vi "Main.vi"() -> ()   [LabVIEW 2017]
uses:
  <vilib>/Platform/TimedLoop/XDataNode/timing_clust.ctl
  <vilib>/Platform/TimedLoop/XDataNode/nitl_modes.ctl
  <vilib>/Platform/TimedLoop/XDataNode/wakeup.ctl
  <vilib>/Analysis/Matrix/Datatypes/RealMatrix.ctl
  <vilib>/Analysis/baseanly.llb/A x Vector.vi
  <vilib>/Analysis/baseanly.llb/Real A x B.vi
  <vilib>/Analysis/_algsub.llb/Real Vector Norm.vi
  <vilib>/Analysis/baseanly.llb/Outer Product.vi
  <vilib>/Analysis/baseanly.llb/Real Outer Product.vi
  <vilib>/robotics/Kinematics/Create Lie Group Matrix.vi
  <vilib>/Analysis/7linalg.llb/Create Special Matrix.vi
  <vilib>/Analysis/7linalg.llb/Create Special Real Matrix.vi
  <vilib>/Analysis/Matrix/Numeric/Multiply/Multiply.vi
  <vilib>/Analysis/Matrix/Numeric/Multiply/Multiply - RM,R.vi
  <vilib>/Analysis/Matrix/Numeric/Multiply/Multiply - R,RM.vi
  <vilib>/Analysis/Matrix/Numeric/Add/Add.vi
  <vilib>/Analysis/Matrix/Numeric/Add/Add - RM,RM.vi
  <vilib>/platform/TimedLoop/XDataNode/XDataNode.xnode
  <vilib>/robotics/Kinematics/NI_Kinematics.lvlib
  <vilib>/Analysis/NI_AALBase.lvlib
  <vilib>/Platform/TimedLoop/XDataNode/XDNodeRunTimeDep.lvlib
  <vilib>/Native 3D Graph/xcontrol/3DPC_SurfacePlot.xctl
  <vilib>/Analysis/Matrix/NI_Matrix.lvlib
  <vilib>/Analysis/NI_AALPro.lvlib
  <vilib>/Native 3D Graph/classes/Base Datatype.lvclass
panel:
  out "policy":dbl[](array[numeric])=[0.3333333333333333, 0.3333333333333333, 0.3333333333333333, 0.3333333333333333, 0.3333333333333333, 0.3333333333333333, 0.3333333333333333, 0.3333333333333333, 0.3333333333333333]
  out "w":dbl[][](array[numeric])
  out "theta":dbl[][](array[numeric])
  out "score":dbl=9.98
  out "break":bool=TRUE
  out "state":dbl[](array[numeric])=[1.3972445388219286, 0.08038206342090427, -148.25832903348876]
  in  "rom":dbl=-45.0
  out "rpy":dbl[](array[numeric])=[inf, inf, inf] format="%#_15g"
  in  "inertia":dbl=1.0
  out "torque":dbl[](array[numeric])
  in  "radius":dbl=1.0
  in  "damping":dbl=0.5
  out "beta2":dbl=0.7460127831658564
  out "v30":dbl[](array[numeric])=[0.5877852522924729, -0.33935797363675174, -0.7344008870614411]
  out "v10":dbl[](array[numeric])=[0.0, 0.6787159472735029, -0.7344008870614411]
  out "v20":dbl[](array[numeric])=[-0.5877852522924731, -0.3393579736367513, -0.7344008870614411]
  out "dt":dbl=0.001
  in  "period":i64=1
  out "v2":dbl[](array[numeric])=[-0.5834154431047975, -0.3393579736367513, -0.7378770808718702]
  out "v1":dbl[](array[numeric])=[0.004359453232169501, 0.6787159472735029, -0.7343879479431492]
  out "v3":dbl[](array[numeric])=[0.5921343495691362, -0.33935797363675174, -0.7308988150144282]
  out "theta":dbl[](array[numeric])=[0.004396877373720295, -0.002202197020422642, -0.002194719520146542] format="%#_15g"
  in  "stop":bool
  out "beta1":dbl=0.9553166181245093
  out "gamma2":dbl=1.2566370614359172
  out "gamma1":dbl=1.5707963267948966
  out "alpha2":dbl=1.5707963267948966
  out "alpha1":dbl=1.5707963267948966
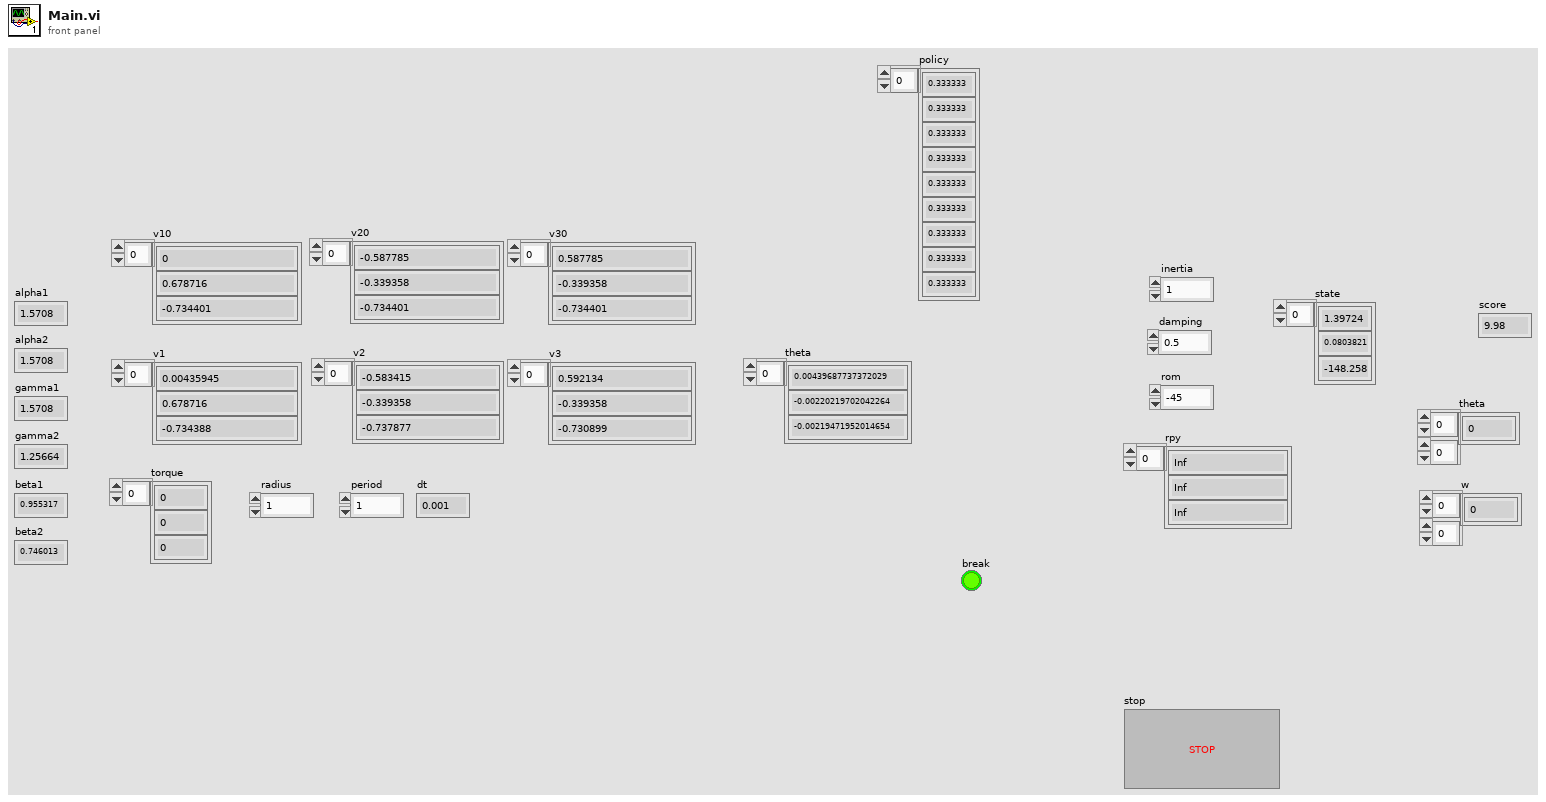
[diagram p1: front panel]
types:
  T1 = typedef "XDNodeRunTimeDep.lvlib/timing_clust.ctl" = cluster{"Expected End [f-1]":u64, "Actual End [f-1]":u64, "Finished Late? [f-1]":bool, "Expected End [i-1]":u64, "Actual End [i-1]":u64, "Finished Late? [i-1]":bool, "Expected Start [i]":u64, "Actual Start [i]":u64, "Expected Start [f]":u64, "Actual Start [f]":u64, "Source Name":string, "Structure Name":string, "Period":i64, "Deadline":i64, "Offset":i64, "Start":i64, "Priority":i32, "Timeout":i32, "Mode":T2, "Wakeup Reason":T3, "Error":errorcluster, "Source Type":string, "Secondary Source Type":string, "Global End Time":u64, "Global Start Time":u64, "Frame Duration":u64, "Iteration Duration":u64, "Assigned CPU":i32, "I/O Scan Engine Mode":u32}
  T2 = typedef "XDNodeRunTimeDep.lvlib/nitl_modes.ctl" = enum32{"No Change", "Process missed periods, maintain original phase", "Discard missed periods, maintain original phase", "Process missed periods, ignore original phase", "Discard missed periods, ignore original phase"}
  T3 = typedef "XDNodeRunTimeDep.lvlib/wakeup.ctl" = enum32{"Normal", "Aborted", "Asynchronous wakeup", "Timing source error", "Timed loop error", "Timeout"}
  T4 = typedef "NI_Matrix.lvlib/RealMatrix.ctl" = dbl[][]
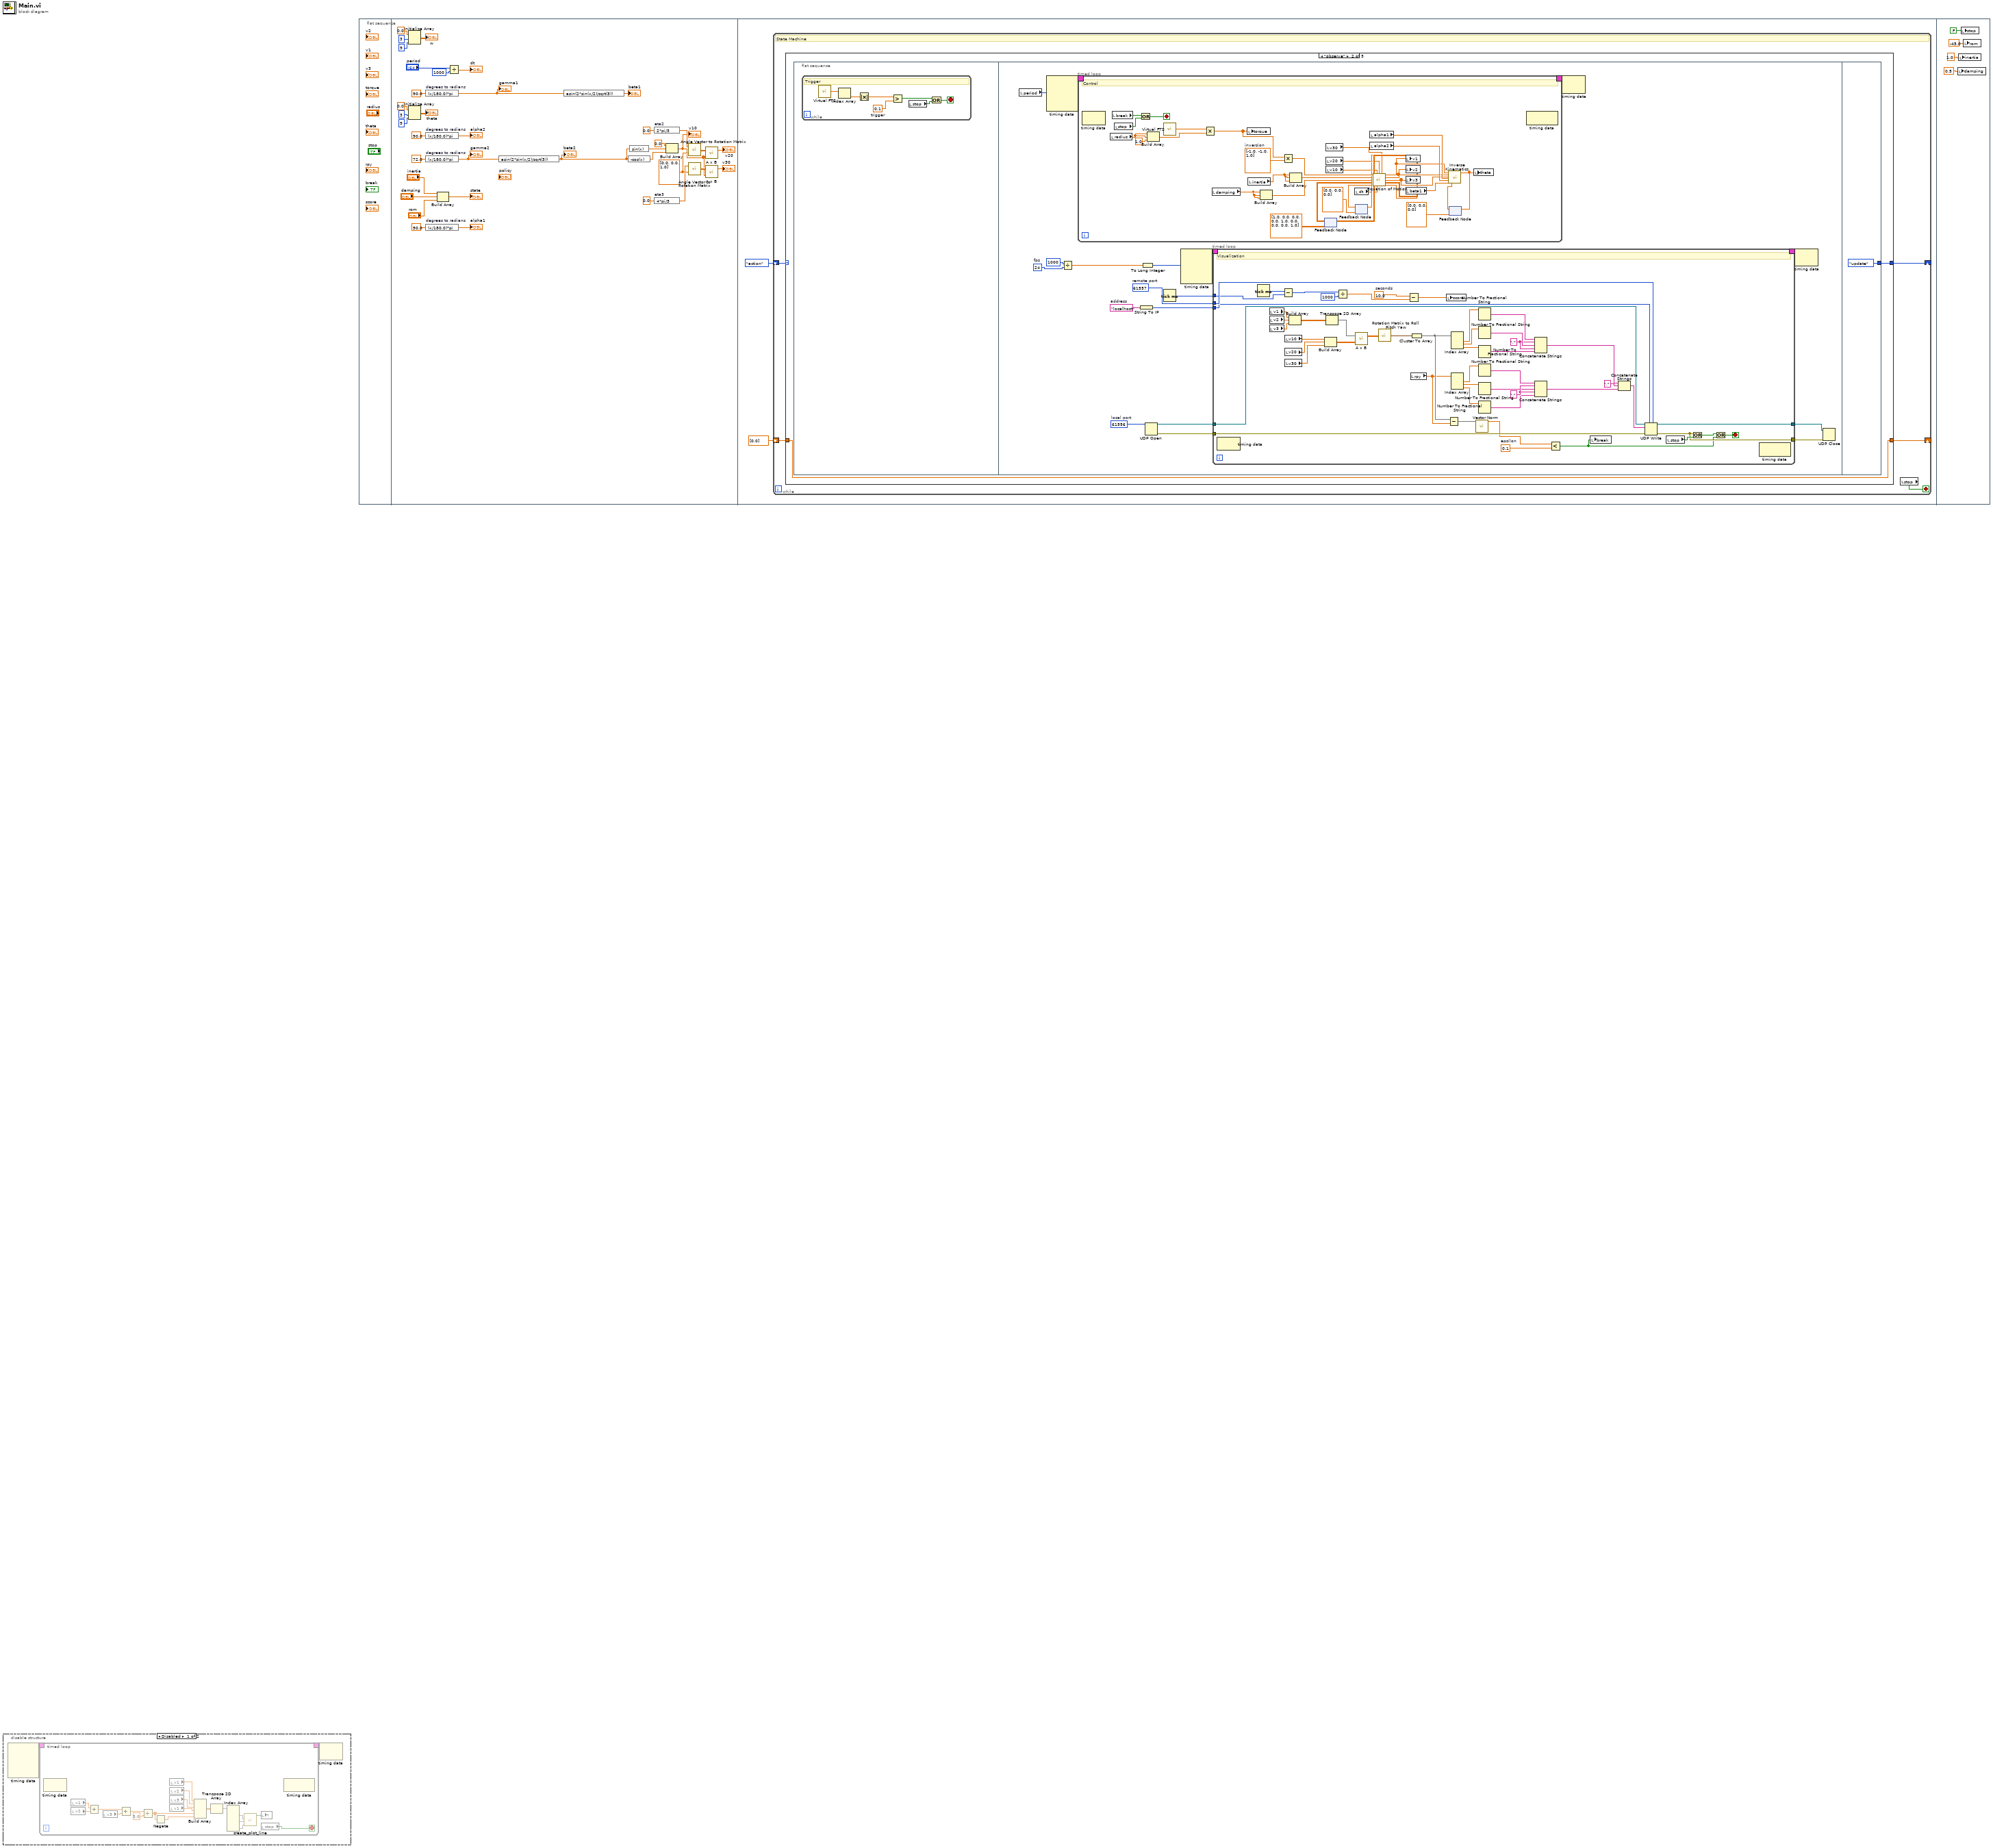
[diagram p0: block diagram]
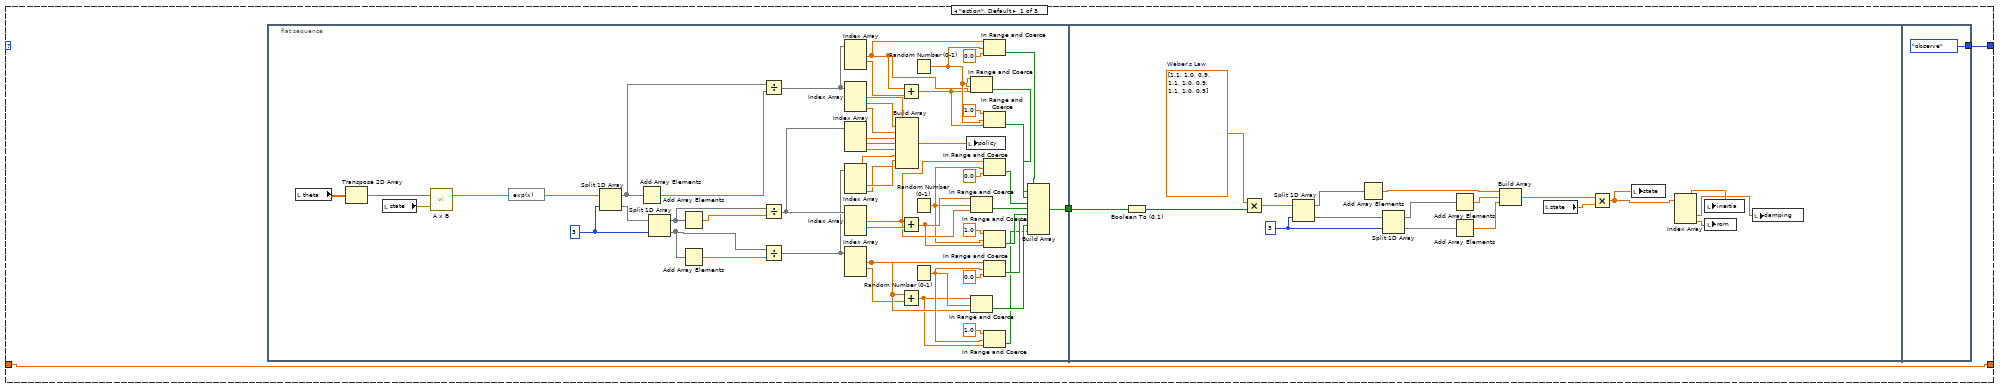
[diagram p3: hidden frame]
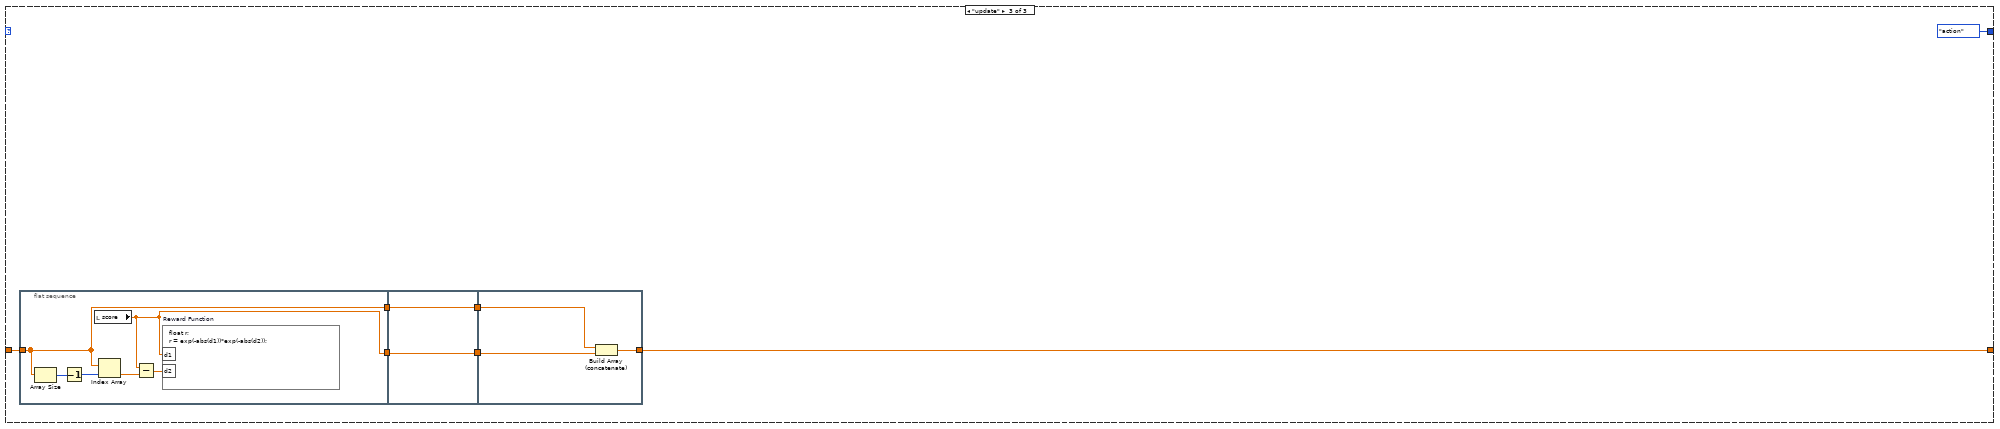
[diagram p4: hidden frame]
diagram:
  n1 = disable-structure shown="Disabled" {
    frame Disabled {
      n2 = node-c288() -> (w2:T1)  [unwired: 4 in]
      n3 = timed-loop {
        timing: w2 -> [_]
        timing-out: [_] -> w1
        stop <- w3 stop-if-true
        n4 = node-c288() -> ()  [unwired: 1 in, 1 out]
        n5 = local read "v1"() -> (w12:dbl[])
        n6 = local read "v2"() -> (w11:dbl[])
        n7 = Add(x=w12, y=w11) -> (x+y=w10:dbl[])
        n8 = local read "v3"() -> (w9:dbl[])
        n9 = Add(x=w10, y=w9) -> (x+y=w8:dbl[])
        n10 = Divide(x=w8, y=3.0) -> (x/y=w6:dbl[])
        n11 = Negate(x=w6) -> (-x=w5:dbl[])
        n12 = local read "v1"() -> (w20:dbl[])
        n13 = local read "v2"() -> (w19:dbl[])
        n14 = local read "v3"() -> (w18:dbl[])
        n15 = local read "v1"() -> (w17:dbl[])
        n16 = Build Array(w20, w19, w18, w17, w6, w5) -> (w16:dbl[][])
        n17 = Transpose 2D Array(2D array=w16) -> (transposed array=w15:dbl[][])
        n18 = Index Array(array=w15) -> (element #1=w14:dbl[], element #2=w13:dbl[], element #3=w4:dbl[])  [unwired: 6 in]
        n19 = call <vilib>:"create_plot_line.vi"("z vector"=w4, "y vector"=w13, "x vector"=w14) -> ("plots out"=w21:refnum<class "Base Datatype.lvclass">[])  [unwired: 2 in, 6 out]
        n20 = local write item#-1(w21) -> ()
        n21 = local read "stop"() -> (w3:bool)
        n22 = node-c288() -> ()  [unwired: 1 in, 1 out]
      }
      n23 = node-c288(w1) -> ()  [unwired: 1 out]
    }
    frame Enabled {
    }
  }
  n24 = flat-sequence {
    frame #0 {
    }
    frame #1 {
      w60 = dbl[] [0.0, 0.0, 1.0] ("vector")
      n25 = Initialize Array(0.0 ("element"), 3 ("dimension size"), 9 ("dimension size")) -> (→"w":dbl[][])
      n26 = Initialize Array(0.0 ("element"), 3 ("dimension size"), 9 ("dimension size")) -> (→"theta":dbl[][])
      n27 = expression code="(x/180.0)*pi" "degrees to radians"(90.0 ("gamma1")) -> (w44:dbl)
      "gamma1" <- w44
      n28 = expression code="(x/180.0)*pi" "degrees to radians"(90.0 ("alpha2")) -> (→"alpha2":dbl)
      n29 = expression code="(x/180.0)*pi" "degrees to radians"(72.0 ("gamma2")) -> (w42:dbl)
      "gamma2" <- w42
      n30 = expression code="(x/180.0)*pi" "degrees to radians"(90.0 ("alpha1")) -> (→"alpha1":dbl)
      n31 = Build Array("inertia", "damping", "rom") -> (→"state":dbl[])
      n32 = Divide(x="period", y=i64 1000) -> (x/y=→"dt":dbl)
      n33 = expression code="asin(2*sin(x/2)/sqrt(3))"(w42) -> (w38:dbl)
      "beta2" <- w38
      n34 = expression code="asin(2*sin(x/2)/sqrt(3))"(w44) -> (→"beta1":dbl)
      n35 = expression code="-cos(x)"(w38) -> (w61:dbl)
      n36 = expression code="sin(x)"(w38) -> (w62:dbl)
      n37 = expression code="2*pi/3" "eta2"(0.0) -> (w59:dbl)
      n38 = expression code="4*pi/3" "eta3"(0.0) -> (w58:dbl)
      n39 = Build Array(0.0 ("element"), w62, w61) -> (w53:dbl[])
      "v10" <- w53
      n40 = call <vilib>:"Angle Vector to Rotation Matrix.vi"("vector"=w60, "angle"=w59) -> ("rotation matrix"=w57:T4)
      n41 = call <vilib>:"Angle Vector to Rotation Matrix.vi"("vector"=w60, "angle"=w58) -> ("rotation matrix"=w56:T4)
      n42 = call-poly <vilib>:"A x B.vi"("Vector"=w53, "A"=w57) -> ("A x Vector"=→"v20":dbl[])  [unwired: 1 out]
      n43 = call-poly <vilib>:"A x B.vi"("Vector"=w53, "A"=w56) -> ("A x Vector"=→"v30":dbl[])  [unwired: 1 out]
    }
    frame #2 {
      # "FK/IK"
      n44 = while {
        shift-right: [w69] -> _
        shift-left: enum16{"action", "observe", "update"}."action" -> [w68]
        shift-right: [w66] -> _
        shift-left: dbl[] [0.0] -> [w67]
        stop <- w70 stop-if-true
        # "State Machine"
        n45 = case shown="\"observe\"" w68 {
          tunnel: [w72 w148 enum16{"action", "observe", "update"}."action"] -> w69
          tunnel: w67 -> [w73 w147 w277]
          tunnel: [w73 w147 w272] -> w66
          frame "action", Default {
            n46 = flat-sequence {
              tunnel: [w87] -> w71
              tunnel: w71 -> [w128]
              tunnel: [enum16{"action", "observe", "update"}."observe"] -> w72
              frame #0 {
                w121 = 3 ("index")
                n47 = local read "theta"() -> (w127:dbl[][])
                n48 = Transpose 2D Array(2D array=w127) -> (transposed array=w126:dbl[][])
                n49 = local read "state"() -> (w125:dbl[])
                n50 = call-poly <vilib>:"A x B.vi"("Vector"=w125, "A"=w126) -> ("A x Vector"=w124:dbl[])  [unwired: 1 out]
                n51 = expression code="exp(x)"(w124) -> (w123:dbl[])
                n52 = Split 1D Array(array=w123, index=w121) -> (first subarray=w119:dbl[], second subarray=w122:dbl[])
                n53 = Add Array Elements(numeric array=w119) -> (sum=w120:dbl)
                n54 = Split 1D Array(array=w122, index=w121) -> (first subarray=w98:dbl[], second subarray=w97:dbl[])
                n55 = Add Array Elements(numeric array=w98) -> (sum=w106:dbl)
                n56 = Add Array Elements(numeric array=w97) -> (sum=w105:dbl)
                n57 = Divide(x=w119, y=w120) -> (x/y=w86:dbl[])
                n58 = Divide(x=w98, y=w106) -> (x/y=w85:dbl[])
                n59 = Divide(x=w97, y=w105) -> (x/y=w84:dbl[])
                n60 = Index Array(array=w86) -> (element #1=w116:dbl, element #2=w115:dbl)  [unwired: 3 in, 1 out]
                n61 = Index Array(array=w86) -> (element #1=w83:dbl, element #2=w82:dbl, element #3=w81:dbl)  [unwired: 3 in]
                n62 = Index Array(array=w85) -> (element #1=w80:dbl, element #2=w79:dbl, element #3=w78:dbl)  [unwired: 3 in]
                n63 = Index Array(array=w84) -> (element #1=w77:dbl, element #2=w76:dbl, element #3=w75:dbl)  [unwired: 3 in]
                n64 = Index Array(array=w85) -> (element #1=w109:dbl, element #2=w110:dbl)  [unwired: 3 in, 1 out]
                n65 = Index Array(array=w84) -> (element #1=w102:dbl, element #2=w101:dbl)  [unwired: 3 in, 1 out]
                n66 = Build Array(w83, w82, w81, w80, w79, w78, w77, w76, w75) -> (w74:dbl[])
                n67 = Add(x=w116, y=w115) -> (x+y=w114:dbl)
                n68 = Add(x=w109, y=w110) -> (x+y=w111:dbl)
                n69 = Add(x=w102, y=w101) -> (x+y=w100:dbl)
                n70 = Random Number (0-1)() -> (number: 0 to 1=w118:dbl)
                n71 = Random Number (0-1)() -> (number: 0 to 1=w107:dbl)
                n72 = Random Number (0-1)() -> (number: 0 to 1=w104:dbl)
                n73 = local write "policy"(w74) -> ()
                n74 = In Range and Coerce(upper limit=w114, x=w118, lower limit=w116) -> (In Range?=w95:bool)  [unwired: 1 out]
                n75 = In Range and Coerce(upper limit=w111, x=w107, lower limit=w109) -> (In Range?=w92:bool)  [unwired: 1 out]
                n76 = In Range and Coerce(upper limit=w100, x=w104, lower limit=w102) -> (In Range?=w89:bool)  [unwired: 1 out]
                n77 = In Range and Coerce(upper limit=w116, x=w118, lower limit=0.0 ("upper limit")) -> (In Range?=w96:bool)  [unwired: 1 out]
                n78 = In Range and Coerce(upper limit=1.0, x=w118, lower limit=w114) -> (In Range?=w94:bool)  [unwired: 1 out]
                n79 = In Range and Coerce(upper limit=w109, x=w107, lower limit=0.0 ("upper limit")) -> (In Range?=w93:bool)  [unwired: 1 out]
                n80 = In Range and Coerce(upper limit=1.0, x=w107, lower limit=w111) -> (In Range?=w91:bool)  [unwired: 1 out]
                n81 = In Range and Coerce(upper limit=w102, x=w104, lower limit=0.0 ("upper limit")) -> (In Range?=w90:bool)  [unwired: 1 out]
                n82 = In Range and Coerce(upper limit=1.0, x=w104, lower limit=w100) -> (In Range?=w88:bool)  [unwired: 1 out]
                n83 = Build Array(w96, w95, w94, w93, w92, w91, w90, w89, w88) -> (w87:bool[])
              }
              frame #1 {
                w135 = 3 ("index")
                w145 = dbl[] [1.1, 1.0, 0.9, 1.1, 1.0, 0.9, 1.1, 1.0, 0.9]  # Weber's Law
                n84 = Boolean To (0,1)(Boolean=w128) -> (0, 1=w144:i16[])
                n85 = Multiply(x=w145, y=w144) -> (x*y=w133:dbl[])
                n86 = Split 1D Array(array=w133, index=w135) -> (first subarray=w136:dbl[], second subarray=w134:dbl[])
                n87 = Add Array Elements(numeric array=w136) -> (sum=w131:dbl)
                n88 = Split 1D Array(array=w134, index=w135) -> (first subarray=w137:dbl[], second subarray=w132:dbl[])
                n89 = Add Array Elements(numeric array=w137) -> (sum=w130:dbl)
                n90 = Add Array Elements(numeric array=w132) -> (sum=w129:dbl)
                n91 = Build Array(w131, w130, w129) -> (w143:dbl[])
                n92 = local read "state"() -> (w142:dbl[])
                n93 = Multiply(x=w143, y=w142) -> (x*y=w141:dbl[])
                n94 = local write "state"(w141) -> ()
                n95 = Index Array(array=w141) -> (element #1=w140:dbl, element #2=w139:dbl, element #3=w138:dbl)  [unwired: 3 in]
                n96 = local write "inertia"(w140) -> ()
                n97 = local write "rom"(w138) -> ()
                n98 = local write "damping"(w139) -> ()
              }
              frame #2 {
              }
            }
          }
          frame "observe" {
            n99 = flat-sequence {
              tunnel: [enum16{"action", "observe", "update"}."update"] -> w148
              frame #0 {
                n100 = while {
                  stop <- w151 stop-if-true
                  w154 = 0.1  # trigger
                  # "Trigger"
                  n101 = call "Virtual FTS.vi"() -> ("value"=w155:dbl[])
                  n102 = Index Array(array=w155) -> (element=w150:dbl)  [unwired: 1 in]
                  n103 = Absolute Value(x=w150) -> (abs(x)=w149:dbl)
                  n104 = Greater?(x=w149, y=w154) -> (0:w153:bool)
                  n105 = local read "stop"() -> (w152:bool)
                  n106 = Or(x=w153, y=w152) -> (x .or. y?=w151:bool)
                }
              }
              frame #1 {
                w162 = 24  # fps
                w164 = "localhost"  # address
                w166 = u16 61557  # remote port
                w169 = u16 61556  # local port
                n107 = local read "period"() -> (w163:i64)
                n108 = node-c288(w163) -> (w173:T1)  [unwired: 3 in]
                n109 = Divide(x=1000, y=w162) -> (x/y=w160:dbl)
                n110 = timed-loop "Timed Loop" {
                  timing: w173 -> [_]
                  timing-out: [_] -> w172
                  stop <- w233 stop-if-true
                  w249 = dbl[] [-1.0, -1.0, 1.0]  # inversion
                  # "Control"
                  n111 = node-c288() -> ()  [unwired: 1 in, 1 out]
                  n112 = local read "radius"() -> (w246:dbl)
                  n113 = local read "break"() -> (w235:bool)
                  n114 = local read "stop"() -> (w234:bool)
                  n115 = Or(x=w235, y=w234) -> (x .or. y?=w233:bool)
                  n116 = Build Array(w246, w246, 1.0 ("element")) -> (w243:dbl[])
                  n117 = call "Virtual FTS.vi"() -> ("value"=w244:dbl[])
                  n118 = Multiply(x=w244, y=w243) -> (x*y=w242:dbl[])
                  n119 = local read "damping"() -> (w231:dbl)
                  n120 = local write "torque"(w242) -> ()
                  n121 = local read "inertia"() -> (w232:dbl)
                  n122 = Build Array(w231, w231, w231) -> (w236:dbl[])
                  n123 = Multiply(x=w242, y=w249) -> (x*y=w250:dbl[])
                  n124 = Build Array(w232, w232, w232) -> (w237:dbl[])
                  n125 = feedback #1(T4 [[1.0, 0.0, 0.0], [0.0, 1.0, 0.0], [0.0, 0.0, 1.0]] ("R'")) -> (w239:T4)
                  n126 = local read "v30"() -> (w251:dbl[])
                  n127 = local read "v20"() -> (w252:dbl[])
                  n128 = local read "v10"() -> (w253:dbl[])
                  n129 = local read "dt"() -> (w241:dbl)
                  n130 = feedback #2(dbl[] [0.0, 0.0, 0.0] ("flow'")) -> (w240:dbl[])
                  n131 = local read "alpha1"() -> (w260:dbl)
                  n132 = local read "alpha2"() -> (w261:dbl)
                  n133 = call "Equation of Motion.vi"("torque"=w250, "v10"=w253, "v20"=w252, "v30"=w251, "inertia"=w237, "damping"=w236, "R"=w239, "omega"=w240, "dt"=w241) -> ("v1d"=w258:dbl[], "v2d"=w257:dbl[], "v3d"=w256:dbl[], "R'"=w255:T4, "omega'"=w248:dbl[])  [unwired: 2 in]
                  n134 = feedback-in #1(w255) -> ()
                  n135 = feedback-in #2(w248) -> ()
                  n136 = local write "v1"(w258) -> ()
                  n137 = local write "v2"(w257) -> ()
                  n138 = local write "v3"(w256) -> ()
                  n139 = local read "beta1"() -> (w262:dbl)
                  n140 = feedback #3(dbl[] [0.0, 0.0, 0.0] ("theta0")) -> (w263:dbl[])
                  n141 = call "Inverse Kinematics.vi"("v1"=w258, "v2"=w257, "v3"=w256, "alpha1"=w260, "alpha2"=w261, "beta1"=w262, "theta"=w263) -> ("theta'"=w259:dbl[])  [unwired: 12 in]
                  n142 = feedback-in #3(w259) -> ()
                  n143 = local write "theta"(w259) -> ()
                  n144 = node-c288() -> ()  [unwired: 1 in, 1 out]
                }
                n145 = String To IP(1:w164) -> (0:w165:u32)
                n146 = To Long Integer(number=w160) -> (32bit integer=w159:i32)
                n147 = UDP Open(11:w169) -> (port=w168:refnum<k16>, 0:w158:errorcluster)  [unwired: 4 in, 1 out]
                n148 = Tick Count (ms)() -> (millisecond timer value=w156:u32)
                n149 = node-c288(w159) -> (w171:T1)  [unwired: 3 in]
                n150 = timed-loop "Timed Loop" {
                  timing: w171 -> [_]
                  timing-out: [_] -> w170
                  tunnel: w168 -> [w224]
                  tunnel: [w223] -> w167
                  tunnel: w166 -> [w215]
                  tunnel: w165 -> [w214]
                  tunnel: w158 -> [w202]
                  tunnel: [w200] -> w157
                  tunnel: w156 -> [w180]
                  stop <- w179 stop-if-true
                  w175 = 10.0  # seconds
                  w184 = 0.1  # epsilon
                  w213 = "," ("string")
                  w216 = "," ("string")
                  # "Visualization"
                  n151 = node-c288() -> ()  [unwired: 1 in, 1 out]
                  n152 = Tick Count (ms)() -> (millisecond timer value=w181:u32)
                  n153 = local read "v1"() -> (w199:dbl[])
                  n154 = local read "v2"() -> (w198:dbl[])
                  n155 = local read "v3"() -> (w197:dbl[])
                  n156 = Subtract(x=w181, y=w180) -> (x-y=w178:u32)
                  n157 = local read "v10"() -> (w194:dbl[])
                  n158 = local read "v20"() -> (w195:dbl[])
                  n159 = local read "v30"() -> (w196:dbl[])
                  n160 = Build Array(w199, w198, w197) -> (w193:dbl[][])
                  n161 = Build Array(w194, w195, w196) -> (w191:dbl[][])
                  n162 = Transpose 2D Array(2D array=w193) -> (transposed array=w192:dbl[][])
                  n163 = Divide(x=w178, y=u32 1000) -> (x/y=w176:dbl)
                  n164 = call-poly <vilib>:"A x B.vi"("B"=w191, "A"=w192) -> ("A x B"=w190:T4)  [unwired: 1 out]
                  n165 = call <vilib>:"Rotation Matrix to Roll Pitch Yaw.vi"("rotation matrix"=w190) -> ("angles"=w189:cluster{"roll":dbl, "pitch":dbl, "yaw":dbl})
                  n166 = Subtract(x=w175, y=w176) -> (x-y=w174:dbl)
                  n167 = Cluster To Array(cluster=w189) -> (array=w188:dbl[])
                  n168 = local read "rpy"() -> (w187:dbl[])
                  n169 = local write "score"(w174) -> ()
                  n170 = Subtract(x=w188, y=w187) -> (x-y=w186:dbl[])
                  n171 = Index Array(array=w188) -> (element #1=w222:dbl, element #2=w221:dbl, element #3=w220:dbl)  [unwired: 3 in]
                  n172 = Index Array(array=w187) -> (element #1=w209:dbl, element #2=w208:dbl, element #3=w207:dbl)  [unwired: 3 in]
                  n173 = call-poly <vilib>:"Vector Norm.vi"("Input Vector"=w186) -> ("norm"=w185:dbl)  [unwired: 9 in, 1 out]
                  n174 = Number To Fractional String(number=w222) -> (F-format string=w219:string)  [unwired: 3 in]
                  n175 = Number To Fractional String(number=w221) -> (F-format string=w218:string)  [unwired: 3 in]
                  n176 = Number To Fractional String(number=w220) -> (F-format string=w217:string)  [unwired: 3 in]
                  n177 = Number To Fractional String(number=w209) -> (F-format string=w210:string)  [unwired: 3 in]
                  n178 = Number To Fractional String(number=w208) -> (F-format string=w211:string)  [unwired: 3 in]
                  n179 = Number To Fractional String(number=w207) -> (F-format string=w212:string)  [unwired: 3 in]
                  n180 = Concatenate Strings(w219, w216, w218, w216, w217) -> (w205:string)
                  n181 = Concatenate Strings(w210, w213, w211, w213, w212) -> (w204:string)
                  n182 = Less?(x=w185, y=w184) -> (x < y?=w182:bool)
                  n183 = local write "break"(w182) -> ()
                  n184 = Concatenate Strings(w205, "," ("string"), w204) -> (w203:string)
                  n185 = UDP Write(address=w214, port or service name=w215, connection ID=w224, data in=w203, 8:w202) -> (error out=w200:errorcluster, 3:w223:refnum<k16>)  [unwired: 1 in]
                  n186 = local read "stop"() -> (w201:bool)
                  n187 = Or(x=w200, y=w201) -> (x .or. y?=w183:bool)
                  n188 = Or(x=w183, y=w182) -> (x .or. y?=w179:bool)
                  n189 = node-c288() -> ()  [unwired: 1 in, 1 out]
                }
                n190 = node-c288(w172) -> ()  [unwired: 1 out]
                n191 = node-c288(w170) -> ()  [unwired: 1 out]
                n192 = UDP Close(connection ID=w167, 8:w157) -> ()  [unwired: 2 out]
              }
              frame #2 {
              }
            }
          }
          frame "update" {
            n193 = flat-sequence {
              tunnel: w277 -> [w279]
              tunnel: [w279] -> w275
              tunnel: [w278] -> w273
              tunnel: [w285] -> w276
              tunnel: w275 -> [w285]
              tunnel: [w284] -> w274
              tunnel: w273 -> [w284]
              tunnel: [w288] -> w272
              tunnel: w276 -> [w287]
              tunnel: w274 -> [w286]
              frame #0 {
                n194 = Array Size(array=w279) -> (size(s)=w282:i32)
                n195 = Decrement(x=w282) -> (x-1=w281:i32)
                n196 = local read "score"() -> (w278:dbl)
                n197 = Index Array(array=w279, index=w281) -> (element=w280:dbl)
                n198 = Subtract(x=w278, y=w280) -> (x-y=w283:dbl)
                n199 = formula code="float r;\nr = exp(-abs(d1))*exp(-abs(d2));" "Reward Function"("d2"=w283, "d1"=w278) -> ()
              }
              frame #1 {
              }
              frame #2 {
                n200 = Build Array (concatenate)(w287, w286) -> (w288:dbl[])
              }
            }
          }
        }
        n201 = local read "stop"() -> (w70:bool)
      }
    }
    frame #3 {
      n202 = local write "damping"(0.5 ("damping (s2)")) -> ()
      n203 = local write "inertia"(1.0 ("inertia (s1)")) -> ()
      n204 = local write "stop"(FALSE ("stop")) -> ()
      n205 = local write "rom"(-45.0 ("rom (s3)")) -> ()
    }
  }
